vi "Crypt_All_Files_In_Hierarchy.vi"(8 "error in (no error)":errorcluster, 10 "Crypting,,,,,,":refnum<vi>, 11 "object in":refnum<class "Crypter.lvclass">) -> (0 "error out":errorcluster, 3 "object out":refnum<class "Crypter.lvclass">)   [LabVIEW 2016, in "Crypter.lvclass"]
uses:
  Crypter.lvclass
  Folder_Mgmt/Folder_Mgmt.lvclass
  C:/Users/Marco Preziani/Documents/DOME-LV16/Crypter/Crypter.lvclass
  Folder_Mgmt/Folder_Mgmt.lvclass/Folder_Mgmt.ctl
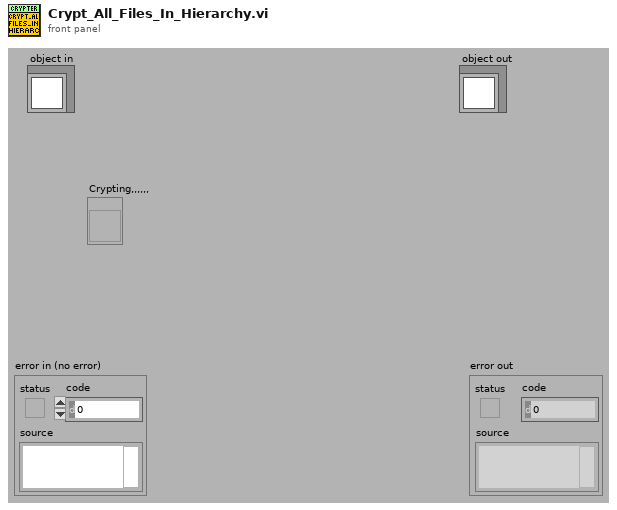
[diagram p1: front panel]
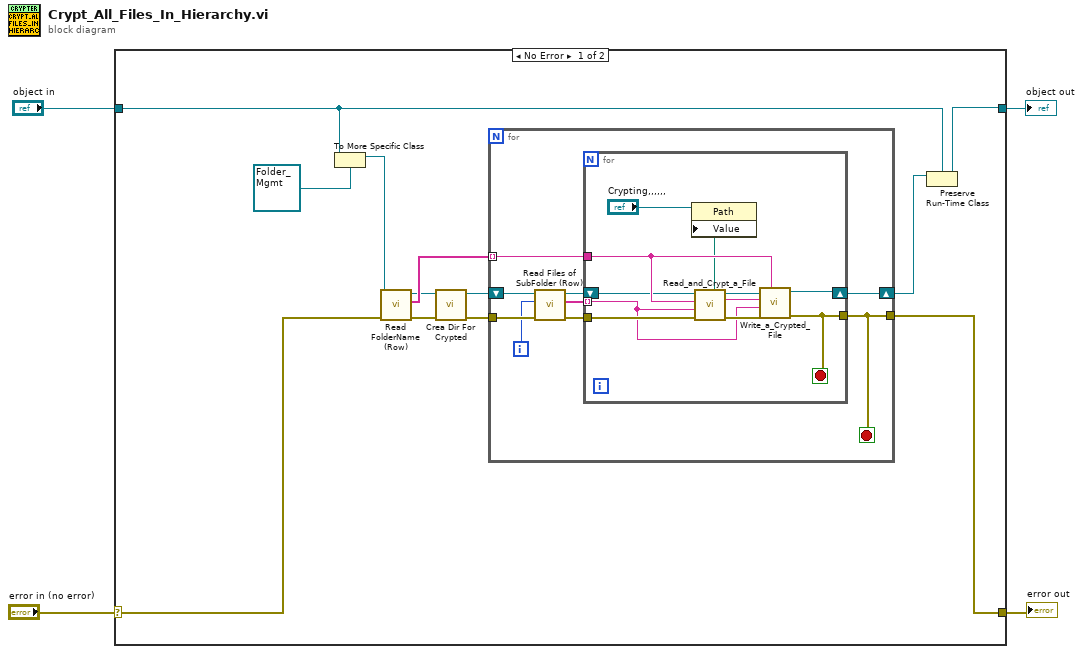
[diagram p0: block diagram]
diagram:
  n1 = case shown="No Error" "error in (no error)" {
    selector: "error in (no error)" -> [w8 w37]
    tunnel: [w14 w37] -> w3
    tunnel: [w6 w36] -> w1
    tunnel: "object in" -> [w7 w36]
    frame No Error {
      n2 = To More Specific Class(target class=refnum<class "Folder_Mgmt.lvclass"> refnum ("Folder_Mgmt.lvclass"), reference=w7) -> (specific class reference=w9:refnum<class "Folder_Mgmt.lvclass">)  [unwired: 1 in, 1 out]
      n3 = call "Read FolderName (Row).vi"("error in (no error)"=w8, "Folder_Mgmt in"=w9) -> ("error out"=w11:errorcluster, "FolderName (Row)"=w15:string[])  [unwired: 7 in, 1 out]
      n4 = call "Crea Dir For Crypted.vi"("error in (no error)"=w11, "Crypter.lvclass"=w9) -> ("error out"=w13:errorcluster, "Crypter.lvclass 2"=w12:refnum<class "Folder_Mgmt.lvclass">)  [unwired: 7 in, 1 out]
      n5 = for {
        tunnel: w15 -> [w19] mode=indexing
        tunnel: w13 -> [w23]
        tunnel: [w18] -> w14
        shift-right: [w16] -> w5
        shift-left: w12 -> [w24]
        i -> [w21]
        stop <- w18 stop-if-true
        n6 = call "Read Files of SubFolder (Row).vi"("error in (no error)"=w23, "RowIndex"=w21, "Folder_Mgmt in"=w24) -> ("error out"=w22:errorcluster, "FolderFiles (Row)"=w20:string[], "Folder_Mgmt out"=w17:refnum<class "Folder_Mgmt.lvclass">)  [unwired: 6 in]
        n7 = for {
          tunnel: w22 -> [w32]
          tunnel: w19 -> [w30]
          tunnel: w20 -> [w31] mode=indexing
          tunnel: [w29] -> w18
          shift-right: [w25] -> w16
          shift-left: w17 -> [w28]
          stop <- w29 stop-if-true
          n8 = call-dynamic "Read_and_Crypt_a_File.vi"("error in (no error)"=w32, "name of File"=w31, "name of Folder"=w30, "object in"=w28) -> ("error out"=w33:errorcluster, "Encrypted text"=w34:string, "object out"=w35:refnum<class "Folder_Mgmt.lvclass">, "Crypting,,,,,,"=w26:path)  [unwired: 4 in]
          n9 = property class="Path"(reference="Crypting,,,,,,", "Value"=w26) -> ()  [unwired: 1 in, 2 out]
          n10 = call-dynamic "Write_a_Crypted_File.vi"("name of Folder"=w30, "error in (no error)"=w33, "name of file"=w31, "Encrypted text"=w34, "object in"=w35) -> ("error out"=w29:errorcluster, "object out"=w25:refnum<class "Folder_Mgmt.lvclass">)  [unwired: 5 in]
        }
      }
      n11 = Preserve Run-Time Class(object in=w5, 2:w7) -> (object out=w6:refnum<class "Crypter.lvclass">)  [unwired: 1 in, 1 out]
    }
    frame Error {
    }
  }
  "error out" <- w3
  "object out" <- w1
